vi "worksheet set vba name.vi"(8 "error in (no error)":errorcluster, 10 "name":string, 11 "worksheet":u32) -> (0 "error out":errorcluster, 3 "function return":u32(ring))   [LabVIEW 2015, in "xlsxwriter.lvlib"]
doc: "lxw_error worksheet_set_vba_name(lxw_worksheet worksheet, const char *name);"
uses:
  xlsxwriter.lvlib
  xlsxwriter.dll
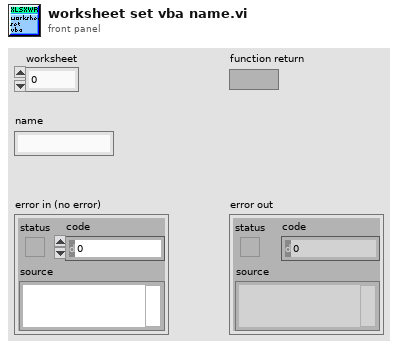
[diagram p1: front panel]
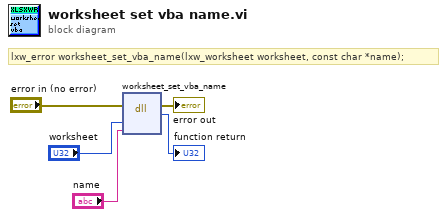
[diagram p0: block diagram]
diagram:
  # "lxw_error worksheet_set_vba_name(lxw_worksheet worksheet, const char *name);"
  n1 = dll-call lib="C:/Users/WDAGUtilityAccount/Desktop/lv_vis_added_cell/xlsxwriter.*" fn="worksheet_set_vba_name"(error in="error in (no error)", "worksheet"="worksheet", "name"="name") -> (error out=→"error out":errorcluster, →"function return":u32)  [unwired: 4 in, 1 out]
